vi "convert--tour to string (chessboard format).vi"(1 "tour":T1[](array[typedef])) -> (0 "tour (chessboard format)":string)   [LabVIEW 2020, in "main.lvlib"]
doc: "Converts the knight tour (array of chessboard_index) to a \"chessboard\" format string."
uses:
  main.lvlib
  core/core_data/chessboard_index.ctl
  core/core_data/core_data.lvlib
panel:
  out "2D array":i32[][](array[numeric])
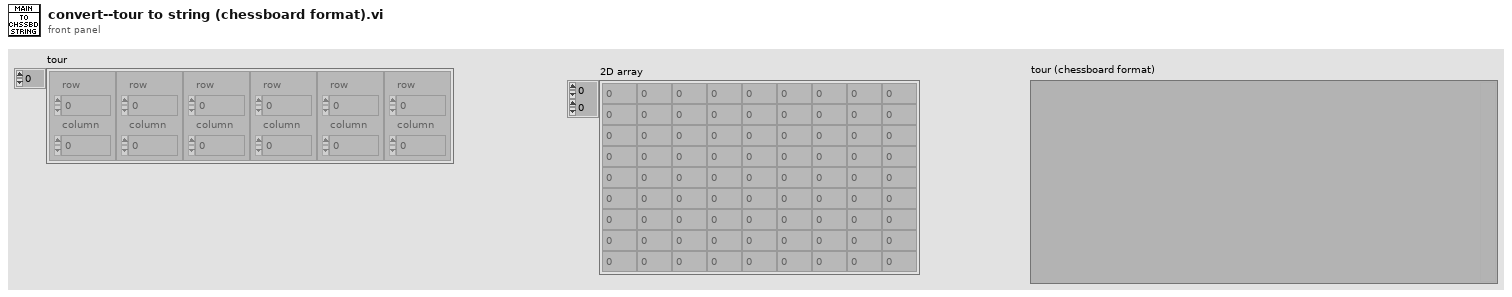
[diagram p1: front panel]
types:
  T1 = typedef "core.lvlib/core_data.lvlib/chessboard_index.ctl" = cluster{"row":u8, "column":u8}
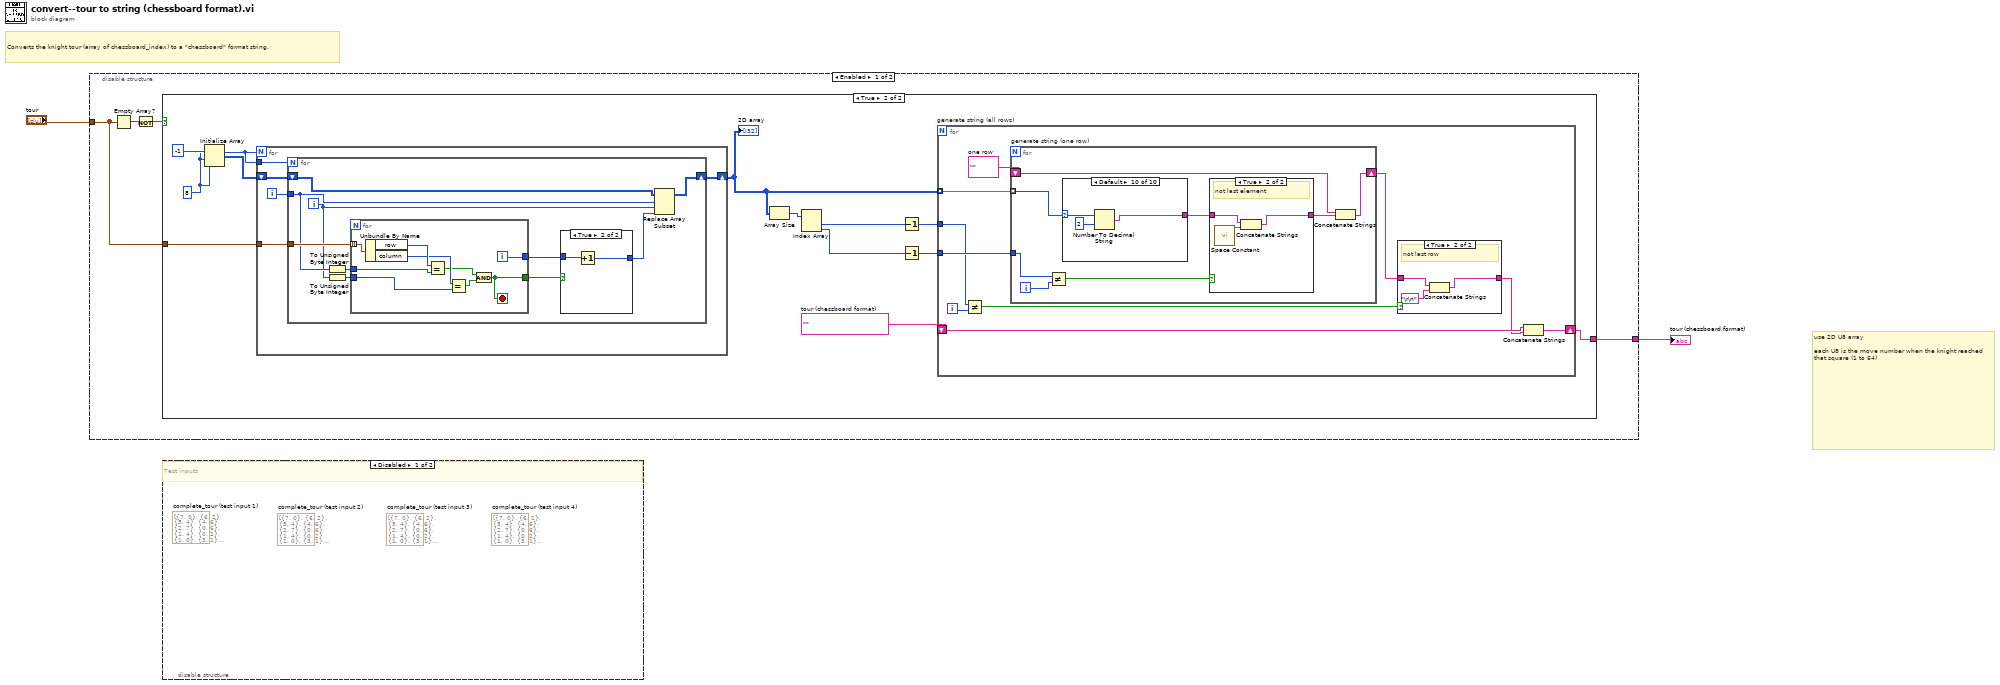
[diagram p0: block diagram]
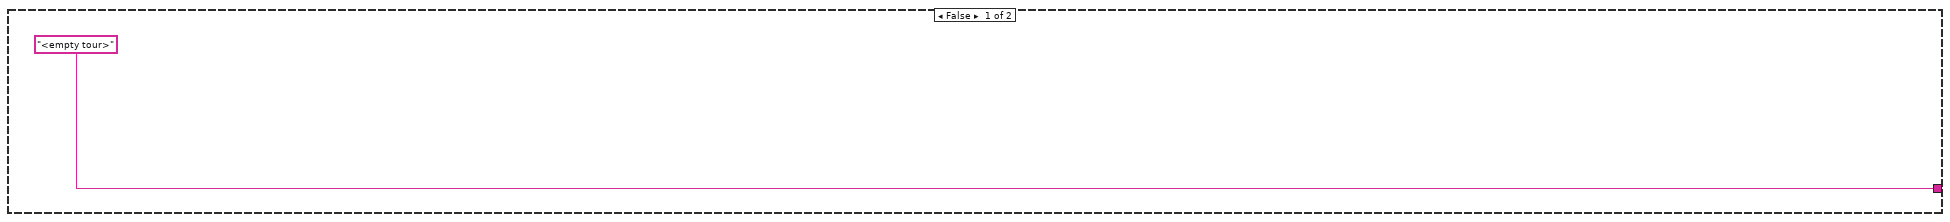
[diagram p2: hidden frame]
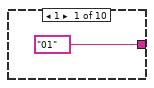
[diagram p5: hidden frame]
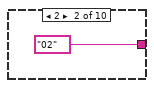
[diagram p6: hidden frame]
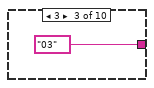
[diagram p7: hidden frame]
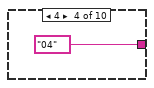
[diagram p8: hidden frame]
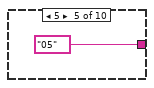
[diagram p9: hidden frame]
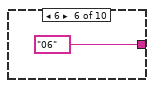
[diagram p10: hidden frame]
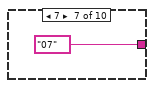
[diagram p11: hidden frame]
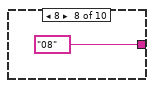
[diagram p12: hidden frame]
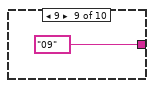
[diagram p13: hidden frame]
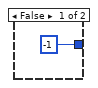
[diagram p14: hidden frame]
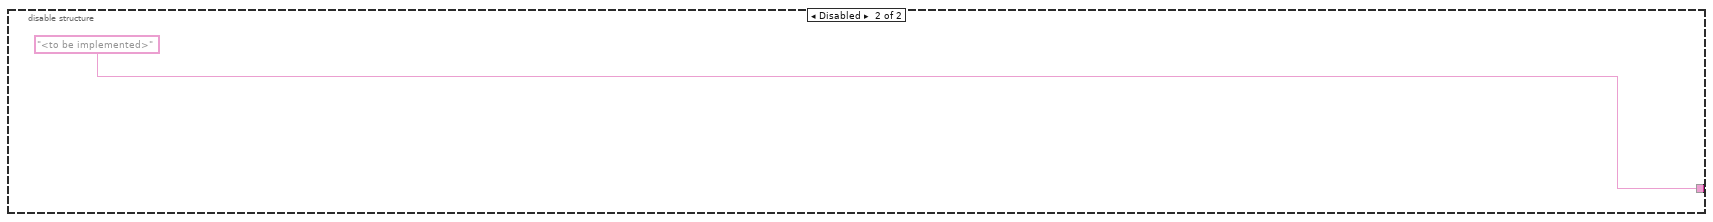
[diagram p15: hidden frame]
diagram:
  # "use 2D U8 array\n\neach U8 is the move number when the knight reached that square (1 to 64)"
  # "Converts the knight tour (array of chessboard_index) to a \"chessboard\" format string."
  n1 = disable-structure shown="Enabled" {
    disable-tunnel: [w4 "<to be implemented>" ("tour (minimalist)")] -> w2
    disable-tunnel: "tour" -> [w3 _]
    frame Enabled {
      n2 = Empty Array?(array=w3) -> (empty?=w6:bool)
      n3 = Not(x=w6) -> (.not. x?=w5:bool)
      n4 = case shown="True" w5 {
        tunnel: ["<empty tour>" w8] -> w4
        tunnel: w3 -> [_ w17]
        frame False {
        }
        frame True {
          w11 = ""  # tour (chessboard format)
          w16 = 8 ("dimension size")
          n5 = Initialize Array(-1, w16, w16) -> (w18:i32[][])
          n6 = for {
            N: w16 -> [_]
            tunnel: w17 -> [w61]
            tunnel: w16 -> [w60]
            shift-right: [w58] -> w15
            shift-left: w18 -> [w62]
            i -> [w59]
            n7 = for {
              N: w60 -> [_]
              tunnel: w61 -> [w71]
              tunnel: w59 -> [w70]
              shift-right: [w63] -> w58
              shift-left: w62 -> [w72]
              i -> [w69]
              n8 = To Unsigned Byte Integer(number=w70) -> (unsigned 8bit integer=w68:u8)
              n9 = To Unsigned Byte Integer(number=w69) -> (unsigned 8bit integer=w67:u8)
              n10 = for {
                tunnel: w71 -> [w84] mode=indexing
                tunnel: w68 -> [w82]
                tunnel: w67 -> [w80]
                tunnel: [w77] -> w66
                tunnel: [w76] -> w65
                i -> [w76]
                stop <- w77 stop-if-true
                n11 = Unbundle By Name(w84) -> ("row"=w83:u8, "column"=w81:u8)
                n12 = Equal?(x=w83, y=w82) -> (x = y?=w78:bool)
                n13 = Equal?(x=w81, y=w80) -> (x = y?=w79:bool)
                n14 = And(x=w78, y=w79) -> (x .and. y?=w77:bool)
              }
              n15 = case shown="True" w66 {
                tunnel: w65 -> [_ w75]
                tunnel: [-1 w74] -> w64
                frame False {
                }
                frame True {
                  n16 = Increment(x=w75) -> (x+1=w74:i32)
                }
              }
              n17 = Replace Array Subset(array=w72, new element=w64, index (row)=w70, index (col)=w69) -> (w63:i32[][])
            }
          }
          "2D array" <- w15
          n18 = Array Size(array=w15) -> (size(s)=w14:i32[])
          n19 = Index Array(array=w14) -> (element #1=w13:i32, element #2=w12:i32)  [unwired: 2 in]
          n20 = Decrement(x=w13) -> (x-1=w10:i32)
          n21 = Decrement(x=w12) -> (x-1=w9:i32)
          n22 = for "generate string (all rows)" {
            tunnel: w15 -> [w29] mode=indexing
            tunnel: w10 -> [w25]
            tunnel: w9 -> [w28]
            shift-right: [w20] -> w8
            shift-left: w11 -> [w22]
            i -> [w26]
            w27 = ""  # one row
            n23 = Not Equal?(x=w25, y=w26) -> (x != y?=w24:bool)
            n24 = for "generate string (one row)" {
              tunnel: w29 -> [w41] mode=indexing
              tunnel: w28 -> [w40]
              shift-right: [w36] -> w23
              shift-left: w27 -> [w35]
              i -> [w39]
              n25 = Not Equal?(x=w40, y=w39) -> (x != y?=w38:bool)
              n26 = case shown="Default" w41 {
                selector: w41 -> [_ _ _ _ _ _ _ _ _ w57]
                tunnel: ["01" "02" "03" "04" "05" "06" "07" "08" "09" w56] -> w37
                frame 1 {
                }
                frame 2 {
                }
                frame 3 {
                }
                frame 4 {
                }
                frame 5 {
                }
                frame 6 {
                }
                frame 7 {
                }
                frame 8 {
                }
                frame 9 {
                }
                frame Default {
                  n27 = Number To Decimal String(number=w57, width (-)=i16 2) -> (decimal integer string=w56:string)
                }
              }
              n28 = case shown="True" w38 {
                tunnel: w37 -> [w42 w45]
                tunnel: [w42 w43] -> w34
                frame False {
                  # "last element"
                }
                frame True {
                  # "not last element"
                  n29 = call <vilib>:"Space Constant.vi"() -> ("String"=w44:string)
                  n30 = Concatenate Strings(w45, w44) -> (w43:string)
                }
              }
              n31 = Concatenate Strings(w35, w34) -> (w36:string)
            }
            n32 = case shown="True" w24 {
              tunnel: w23 -> [w30 w33]
              tunnel: [w30 w31] -> w21
              frame False {
                # "last row"
              }
              frame True {
                # "not last row"
                n33 = Concatenate Strings(w33, "\r\n") -> (w31:string)
              }
            }
            n34 = Concatenate Strings(w22, w21) -> (w20:string)
          }
        }
      }
    }
    frame Disabled {
    }
  }
  "tour (chessboard format)" <- w2
  n35 = disable-structure shown="Disabled" {
    frame Disabled {
      (unwired) T1[] [{"row"=7, "column"=0}, {"row"=6, "column"=2}, {"row"=5, "column"=4}, {"row"=4, "column"=6}, {"row"=2, "column"=7}, {"row"=0, "column"=6}, {"row"=1, "column"=4}, {"row"=0, "column"=2}, {"row"=1, "column"=0}, {"row"=3, "column"=1}, {"row"=2, "column"=3}, {"row"=1, "column"=5}, {"row"=0, "column"=7}, {"row"=2, "column"=6}, {"row"=0, "column"=5}, {"row"=1, "column"=3}, {"row"=0, "column"=1}, {"row"=2, "column"=0}, {"row"=1, "column"=2}, {"row"=0, "column"=4}, {"row"=2, "column"=5}, {"row"=1, "column"=7}, {"row"=3, "column"=6}, {"row"=2, "column"=4}, {"row"=1, "column"=6}, {"row"=3, "column"=5}, {"row"=4, "column"=3}, {"row"=2, "column"=2}, {"row"=0, "column"=3}, {"row"=1, "column"=1}, {"row"=3, "column"=0}, {"row"=5, "column"=1}, {"row"=7, "column"=2}, {"row"=6, "column"=4}, {"row"=7, "column"=6}, {"row"=5, "column"=7}, {"row"=4, "column"=5}, {"row"=3, "column"=7}, {"row"=5, "column"=6}, {"row"=7, "column"=7}, {"row"=6, "column"=5}, {"row"=7, "column"=3}, {"row"=6, "column"=1}, {"row"=4, "column"=0}, {"row"=3, "column"=2}, {"row"=4, "column"=4}, {"row"=6, "column"=3}, {"row"=7, "column"=5}, {"row"=6, "column"=7}, {"row"=5, "column"=5}, {"row"=4, "column"=7}, {"row"=6, "column"=6}, {"row"=7, "column"=4}, {"row"=5, "column"=3}, {"row"=3, "column"=4}, {"row"=4, "column"=2}, {"row"=5, "column"=0}, {"row"=7, "column"=1}, {"row"=5, "column"=2}, {"row"=6, "column"=0}, {"row"=4, "column"=1}, {"row"=3, "column"=3}, {"row"=2, "column"=1}, {"row"=0, "column"=0}]  # complete_tour (test input 4)
      (unwired) T1[] [{"row"=7, "column"=0}, {"row"=6, "column"=2}, {"row"=5, "column"=4}, {"row"=4, "column"=6}, {"row"=2, "column"=7}, {"row"=0, "column"=6}, {"row"=1, "column"=4}, {"row"=0, "column"=2}, {"row"=1, "column"=0}, {"row"=3, "column"=1}, {"row"=2, "column"=3}, {"row"=1, "column"=5}, {"row"=0, "column"=7}, {"row"=2, "column"=6}, {"row"=0, "column"=5}, {"row"=1, "column"=3}, {"row"=0, "column"=1}, {"row"=2, "column"=0}, {"row"=1, "column"=2}, {"row"=0, "column"=4}, {"row"=2, "column"=5}, {"row"=1, "column"=7}, {"row"=3, "column"=6}, {"row"=2, "column"=4}, {"row"=1, "column"=6}, {"row"=3, "column"=5}, {"row"=4, "column"=3}, {"row"=2, "column"=2}, {"row"=0, "column"=3}, {"row"=1, "column"=1}, {"row"=3, "column"=0}, {"row"=5, "column"=1}, {"row"=3, "column"=2}, {"row"=4, "column"=4}, {"row"=6, "column"=3}, {"row"=7, "column"=5}, {"row"=6, "column"=7}, {"row"=5, "column"=5}, {"row"=4, "column"=7}, {"row"=6, "column"=6}, {"row"=7, "column"=4}, {"row"=5, "column"=3}, {"row"=3, "column"=4}, {"row"=4, "column"=2}, {"row"=5, "column"=0}, {"row"=7, "column"=1}, {"row"=5, "column"=2}, {"row"=4, "column"=0}, {"row"=6, "column"=1}, {"row"=7, "column"=3}, {"row"=6, "column"=5}, {"row"=7, "column"=7}, {"row"=5, "column"=6}, {"row"=3, "column"=7}, {"row"=4, "column"=5}, {"row"=5, "column"=7}, {"row"=7, "column"=6}, {"row"=6, "column"=4}, {"row"=7, "column"=2}, {"row"=6, "column"=0}, {"row"=4, "column"=1}, {"row"=3, "column"=3}, {"row"=2, "column"=1}, {"row"=0, "column"=0}]  # complete_tour (test input 3)
      (unwired) T1[] [{"row"=7, "column"=0}, {"row"=6, "column"=2}, {"row"=5, "column"=4}, {"row"=4, "column"=6}, {"row"=2, "column"=7}, {"row"=0, "column"=6}, {"row"=1, "column"=4}, {"row"=0, "column"=2}, {"row"=1, "column"=0}, {"row"=3, "column"=1}, {"row"=2, "column"=3}, {"row"=1, "column"=5}, {"row"=0, "column"=7}, {"row"=2, "column"=6}, {"row"=0, "column"=5}, {"row"=1, "column"=3}, {"row"=0, "column"=1}, {"row"=2, "column"=0}, {"row"=1, "column"=2}, {"row"=0, "column"=4}, {"row"=2, "column"=5}, {"row"=1, "column"=7}, {"row"=3, "column"=6}, {"row"=2, "column"=4}, {"row"=1, "column"=6}, {"row"=3, "column"=5}, {"row"=4, "column"=3}, {"row"=2, "column"=2}, {"row"=0, "column"=3}, {"row"=1, "column"=1}, {"row"=3, "column"=0}, {"row"=5, "column"=1}, {"row"=3, "column"=2}, {"row"=4, "column"=4}, {"row"=6, "column"=3}, {"row"=7, "column"=5}, {"row"=6, "column"=7}, {"row"=5, "column"=5}, {"row"=4, "column"=7}, {"row"=6, "column"=6}, {"row"=7, "column"=4}, {"row"=5, "column"=3}, {"row"=3, "column"=4}, {"row"=4, "column"=2}, {"row"=5, "column"=0}, {"row"=7, "column"=1}, {"row"=5, "column"=2}, {"row"=3, "column"=3}, {"row"=4, "column"=1}, {"row"=6, "column"=0}, {"row"=7, "column"=2}, {"row"=6, "column"=4}, {"row"=7, "column"=6}, {"row"=5, "column"=7}, {"row"=4, "column"=5}, {"row"=3, "column"=7}, {"row"=5, "column"=6}, {"row"=7, "column"=7}, {"row"=6, "column"=5}, {"row"=7, "column"=3}, {"row"=6, "column"=1}, {"row"=4, "column"=0}, {"row"=2, "column"=1}, {"row"=0, "column"=0}]  # complete_tour (test input 2)
      (unwired) T1[] [{"row"=7, "column"=0}, {"row"=6, "column"=2}, {"row"=5, "column"=4}, {"row"=4, "column"=6}, {"row"=2, "column"=7}, {"row"=0, "column"=6}, {"row"=1, "column"=4}, {"row"=0, "column"=2}, {"row"=1, "column"=0}, {"row"=3, "column"=1}, {"row"=2, "column"=3}, {"row"=1, "column"=5}, {"row"=0, "column"=7}, {"row"=2, "column"=6}, {"row"=0, "column"=5}, {"row"=1, "column"=3}, {"row"=0, "column"=1}, {"row"=2, "column"=0}, {"row"=1, "column"=2}, {"row"=0, "column"=4}, {"row"=2, "column"=5}, {"row"=1, "column"=7}, {"row"=3, "column"=6}, {"row"=2, "column"=4}, {"row"=1, "column"=6}, {"row"=3, "column"=5}, {"row"=4, "column"=3}, {"row"=2, "column"=2}, {"row"=0, "column"=3}, {"row"=1, "column"=1}, {"row"=3, "column"=0}, {"row"=5, "column"=1}, {"row"=3, "column"=2}, {"row"=4, "column"=0}, {"row"=6, "column"=1}, {"row"=7, "column"=3}, {"row"=5, "column"=2}, {"row"=7, "column"=1}, {"row"=5, "column"=0}, {"row"=4, "column"=2}, {"row"=3, "column"=4}, {"row"=5, "column"=3}, {"row"=7, "column"=4}, {"row"=6, "column"=6}, {"row"=4, "column"=7}, {"row"=5, "column"=5}, {"row"=6, "column"=7}, {"row"=7, "column"=5}, {"row"=6, "column"=3}, {"row"=4, "column"=4}, {"row"=6, "column"=5}, {"row"=7, "column"=7}, {"row"=5, "column"=6}, {"row"=3, "column"=7}, {"row"=4, "column"=5}, {"row"=5, "column"=7}, {"row"=7, "column"=6}, {"row"=6, "column"=4}, {"row"=7, "column"=2}, {"row"=6, "column"=0}, {"row"=4, "column"=1}, {"row"=3, "column"=3}, {"row"=2, "column"=1}, {"row"=0, "column"=0}]  # complete_tour (test input 1)
      # "Test inputs"
    }
    frame Enabled {
    }
  }
